vi "GetTableName.vi"(8 "error in (no error)":errorcluster, 11 "TMflexDatabase in":refnum<class "TMflexDatabase.lvclass">) -> (0 "error out":errorcluster, 2 "TableName":string, 3 "TMflexDatabase out":refnum<class "TMflexDatabase.lvclass">)   [LabVIEW 2015, in "TMflexDatabase.lvclass"]
uses:
  TMflexDatabase.lvclass
  TMflexDatabase.lvclass/TMflexDatabase.ctl
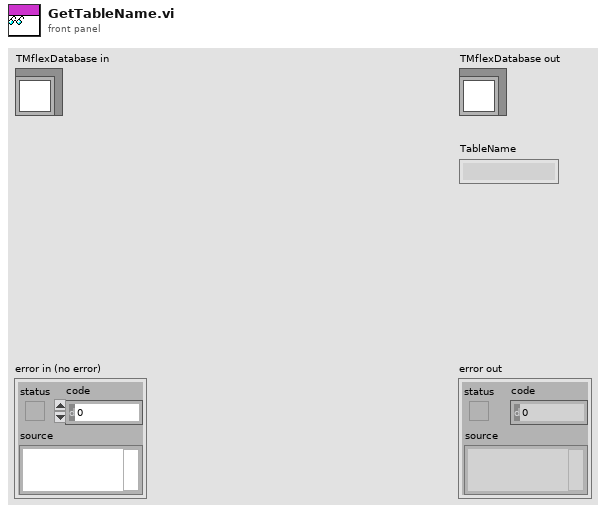
[diagram p1: front panel]
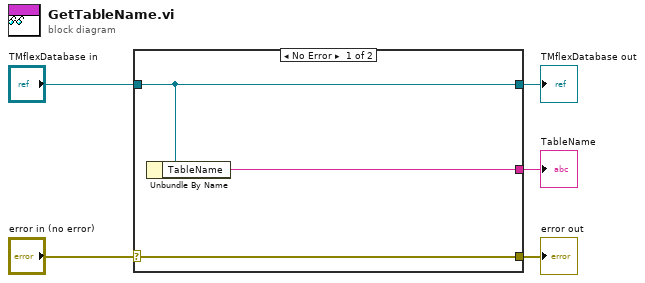
[diagram p0: block diagram]
diagram:
  n1 = case shown="No Error" "error in (no error)" {
    selector: "error in (no error)" -> [w8 w9]
    tunnel: [w8 w9] -> w4
    tunnel: [w7 w10] -> w2
    tunnel: "TMflexDatabase in" -> [w7 w10]
    tunnel: [w6 _] -> w1
    frame No Error {
      n2 = Unbundle By Name(w7) -> ("TableName"=w6:string)
    }
    frame Error {
    }
  }
  "error out" <- w4
  "TMflexDatabase out" <- w2
  "TableName" <- w1
